vi "T_sat_correlation.vi"(0 "P [Pa]":dbl) -> (1 "T Sat [C]":dbl, 2 "formula":string="-111.391+27.3512*ln(x/1000)  ")   [LabVIEW 2017]
uses:
  <vilib>/gmath/NI_Gmath.lvlib
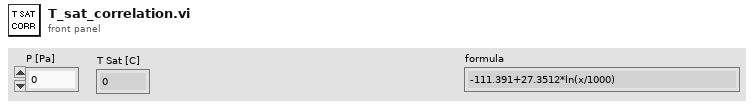
[diagram p1: front panel]
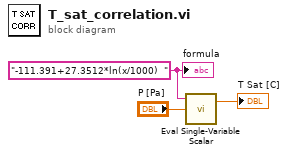
[diagram p0: block diagram]
diagram:
  w3 = "-111.391+27.3512*ln(x/1000)  " ("formula")
  n1 = call <vilib>:"Eval Single-Variable Scalar.vi"("x value"="P [Pa]", "formula"=w3) -> ("y value"=→"T Sat [C]":dbl)  [unwired: 1 in, 1 out]
  "formula" <- w3
